vi "Configure Load to Sequence - ganged.vi"(8 "error in":errorcluster, 10 "measurement configuration":T6 {"Measurement timeout" format="%.3p"; "Load device voltage/current rating" format="%#_6pA"; "Load voltage/current setpoints" format="%#_6p"; "Load output function" items=["DC Voltage"=1006, "DC Current"=1007, "Pulse Voltage"=1049, "Pulse Current"=1050]; "Load sense" items=["Local"=1008, "Remote"=1009]; "Load transient response" items=["Slow"=1041, "Normal"=1038, "Fast"=1039, "Custom"=1042]; "Load current/voltage limit high" format="%#_6p"; "Load current/voltage limit low" format="%#_6p"; "Load current/voltage limit range" format="%#_6p"; "Load voltage/current level range" format="%#_6p"; "Power ON/Source voltage/current setpoints" format="%#_6p"; "Power ON/Source output function" items=["DC Voltage"=1006, "DC Current"=1007, "Pulse Voltage"=1049, "Pulse Current"=1050]; "Power ON/Source sense" items=["Local"=1008, "Remote"=1009]; "Source transient response" items=["Slow"=1041, "Normal"=1038, "Fast"=1039, "Custom"=1042]; "Source current/voltage limit high" format="%#_6p"; "Source current/voltage limit low" format="%#_6p"; "Power ON/Source current/voltage limit range" format="%#_6p"; "Source voltage/current level range" format="%#_6p"}, 11 "Waveform Mode - Control":T1={"Source Ganged Session Out"={"Ganged Config"=enum."Series", "Session List"=[], "Session Mode"=[], "Channel"=[]}, "Load Ganged Session Out"={"Ganged Config"=enum."Series", "Session List"=[], "Session Mode"=[], "Channel"=[]}, "Source Measure Record Length"=0, "Load Measure Record Length"=0, "Source Sequence Name"="", "Load Sequence Name"="", "Source First Sequence Call"=FALSE, "Load First Sequence Call"=FALSE, "Measurement Results"={"Source dt"=[], "Source voltages"=[], "Source currents"=[], "Ganged source voltages"=[], "Ganged source currents"=[0.0], "Load dt"=[], "Load voltages"=[], "Load currents"=[], "Ganged load voltages"=[], "Ganged load currents"=[], "Status"="", "Eload status"=""}, "No. of eload used"=0, "Measurement timeout"=0.0, "Load Source ON/OFF"=enum."SOURCE AND LOAD ON", "Load session out"="", "Source session out"="", "Load channel name"="", "Source channel name"="", "Source ganged/single"=FALSE, "Load ganged/single"=FALSE, "Source Master/Single resource name"="", "Source Slave resource name"=[], "Load Master/Single resource name"="", "Load Slave resource name"=[]}) -> (0 "error out":errorcluster, 3 "Waveform Mode - Result":T1={"Source Ganged Session Out"={"Ganged Config"=enum."Series", "Session List"=[], "Session Mode"=[], "Channel"=[]}, "Load Ganged Session Out"={"Ganged Config"=enum."Series", "Session List"=[], "Session Mode"=[], "Channel"=[]}, "Source Measure Record Length"=0, "Load Measure Record Length"=0, "Source Sequence Name"="", "Load Sequence Name"="", "Source First Sequence Call"=FALSE, "Load First Sequence Call"=FALSE, "Measurement Results"={"Source dt"=[], "Source voltages"=[], "Source currents"=[], "Ganged source voltages"=[], "Ganged source currents"=[0.0], "Load dt"=[], "Load voltages"=[], "Load currents"=[], "Ganged load voltages"=[], "Ganged load currents"=[], "Status"="", "Eload status"=""}, "No. of eload used"=0, "Measurement timeout"=0.0, "Load Source ON/OFF"=enum."SOURCE AND LOAD ON", "Load session out"="", "Source session out"="", "Load channel name"="", "Source channel name"="", "Source ganged/single"=FALSE, "Load ganged/single"=FALSE, "Source Master/Single resource name"="", "Source Slave resource name"=[], "Load Master/Single resource name"="", "Load Slave resource name"=[]})   [LabVIEW 2021, in "Waveform Mode_Channel Ganging.lvlib"]
doc: "Configures load ganged to sequence"
uses:
  Measurement Configuration.ctl
  Controls/Waveform Mode Measurement.ctl
  shared subVIs/ctl/NIDCPower_channel_ganging - ctl - ganged session.ctl
  shared subVIs/ctl/NIDCPower_channel_ganging - ctl - ganged config.ctl
  shared subVIs/ctl/NIDCPower_channel_ganging - ctl - channel mode.ctl
  Measurement Results.ctl
  <instrlib>/niDCPower/nidcpower.llb/niDCPower Source Mode.ctl
  <instrlib>/niDCPower/nidcpower.llb/niDCPower Sequence Attribute Type.ctl
  <instrlib>/niDCPower/nidcpower.llb/niDCPower Create Advanced Sequence Step With Channels.vi
  Waveform Mode_Channel Ganging.lvlib
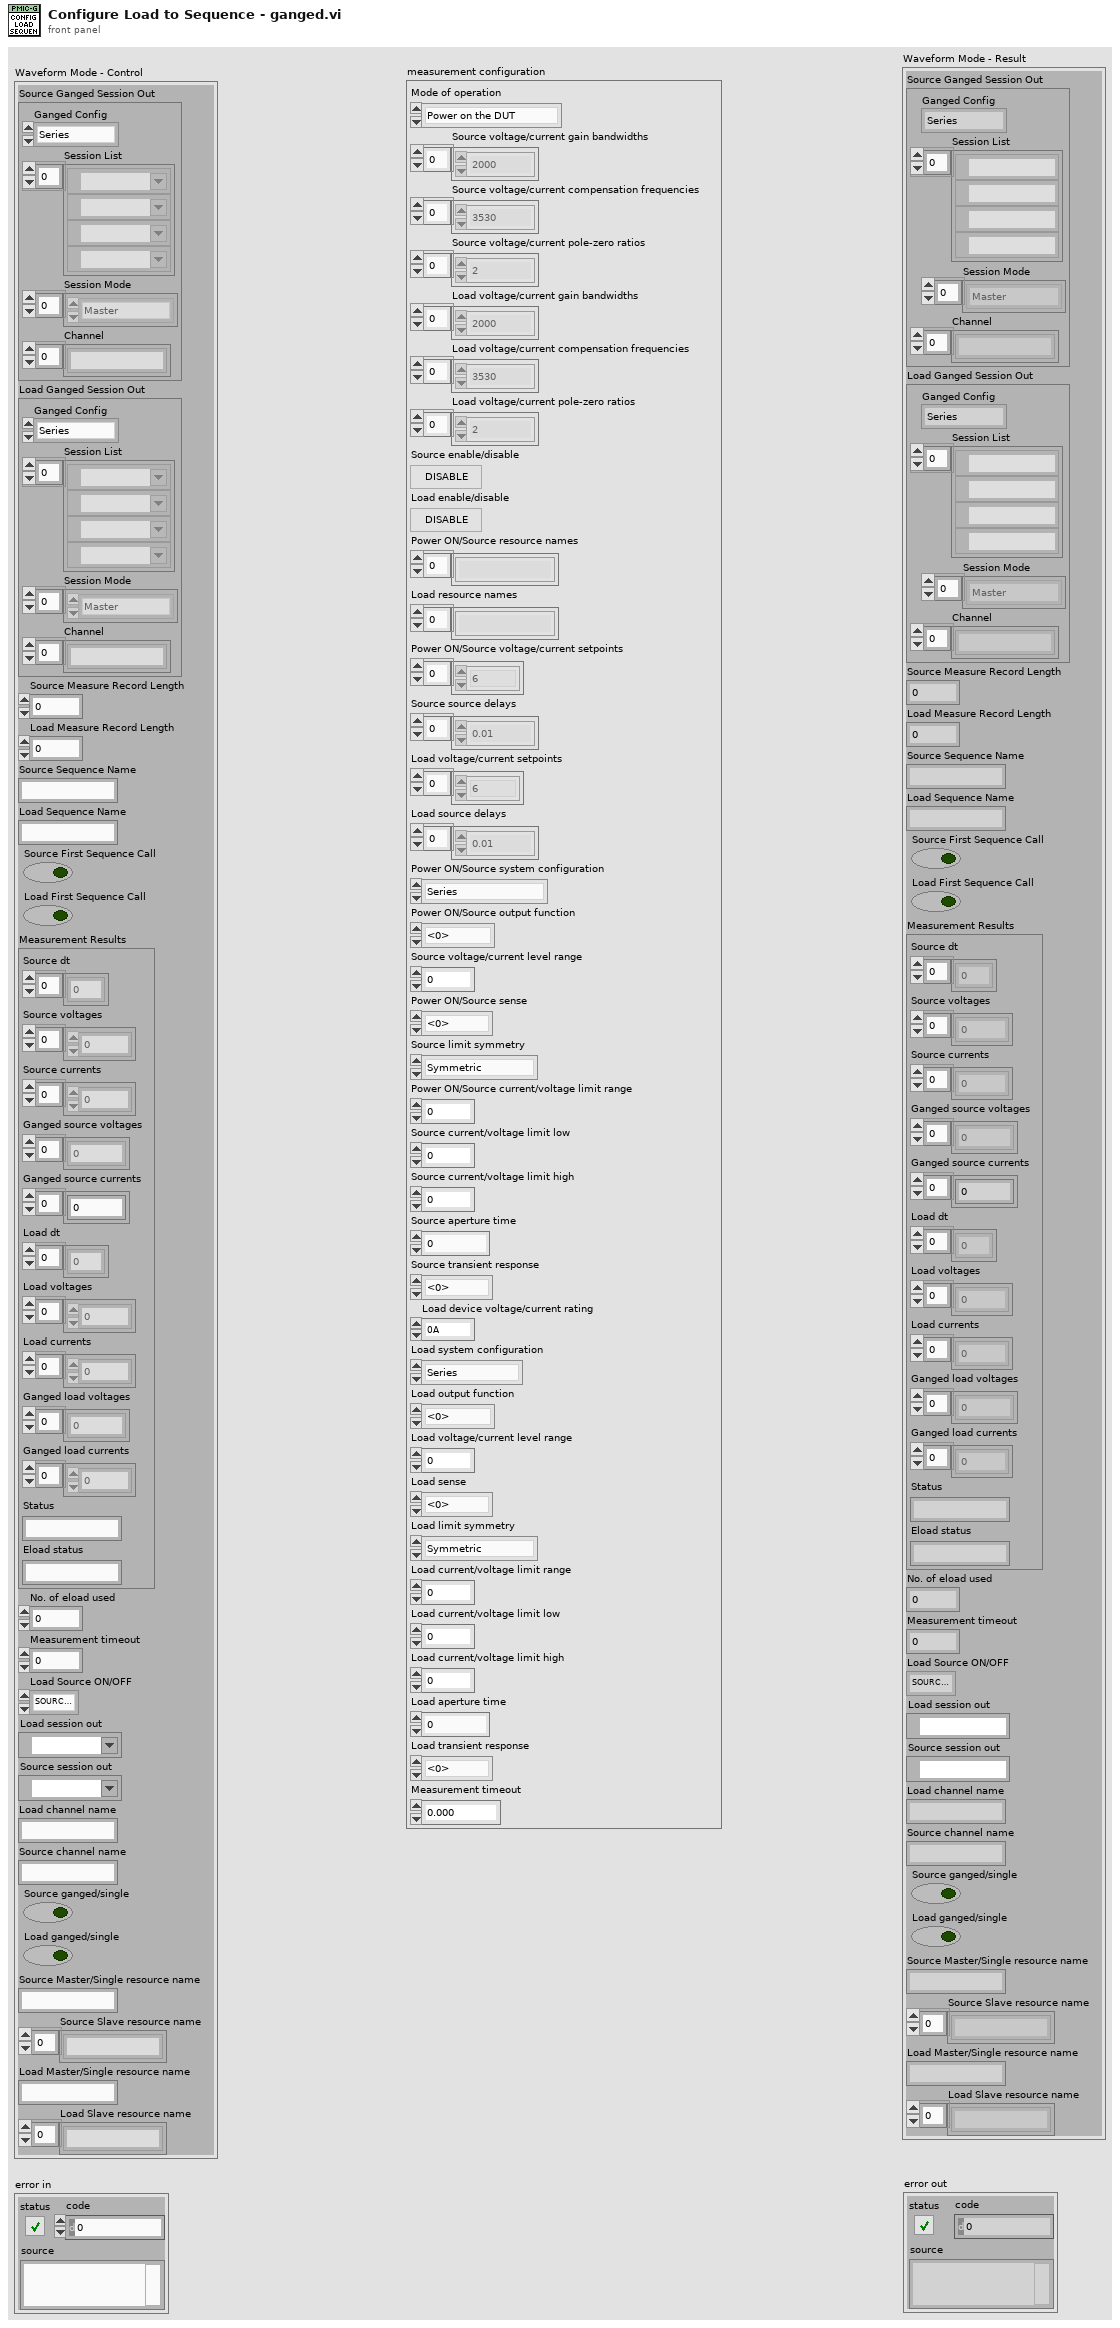
[diagram p1: front panel]
types:
  T1 = typedef "Waveform Mode_Channel Ganging.lvlib/Waveform Mode Measurement.ctl" = cluster{"Source Ganged Session Out":T2, "Load Ganged Session Out":T2, "Source Measure Record Length":i32, "Load Measure Record Length":i32, "Source Sequence Name":string, "Load Sequence Name":string, "Source First Sequence Call":bool, "Load First Sequence Call":bool, "Measurement Results":T5, "No. of eload used":i32, "Measurement timeout":dbl, "Load Source ON/OFF":enum16{"SOURCE AND LOAD OFF", "SOURCE ON", "LOAD ON", "SOURCE AND LOAD ON"}, "Load session out":refnum<k15>, "Source session out":refnum<k15>, "Load channel name":string, "Source channel name":string, "Source ganged/single":bool, "Load ganged/single":bool, "Source Master/Single resource name":string, "Source Slave resource name":string[], "Load Master/Single resource name":string, "Load Slave resource name":string[]}
  T2 = typedef "NIDCPower_channel_ganging - ctl - ganged session.ctl" = cluster{"Ganged Config":T3, "Session List":refnum<k15>[], "Session Mode":T4[], "Channel":string[]}
  T3 = typedef "NIDCPower_channel_ganging - ctl - ganged config.ctl" = enum32{"Series", "Parallel", "Manual"}
  T4 = typedef "NIDCPower_channel_ganging - ctl - channel mode.ctl" = enum32{"Master", "Slave", "Slave - Inverted"}
  T5 = typedef "Waveform Mode_Channel Ganging.lvlib/Measurement Results.ctl" = cluster{"Source dt":dbl[], "Source voltages":dbl[], "Source currents":dbl[], "Ganged source voltages":dbl[], "Ganged source currents":dbl[], "Load dt":dbl[], "Load voltages":dbl[], "Load currents":dbl[], "Ganged load voltages":dbl[], "Ganged load currents":dbl[], "Status":string, "Eload status":string}
  T6 = typedef "Waveform Mode_Channel Ganging.lvlib/Measurement Configuration.ctl" = cluster{"Mode of operation":enum32{"Power on the DUT", "Perform measurement", "Power off the DUT"}, "Source voltage/current gain bandwidths":dbl[], "Source voltage/current compensation frequencies":dbl[], "Source voltage/current pole-zero ratios":dbl[], "Load voltage/current gain bandwidths":dbl[], "Load voltage/current compensation frequencies":dbl[], "Load voltage/current pole-zero ratios":dbl[], "Source enable/disable":bool, "Load enable/disable":bool, "Power ON/Source resource names":string[], "Load resource names":string[], "Power ON/Source voltage/current setpoints":dbl[], "Source source delays":dbl[], "Load voltage/current setpoints":dbl[], "Load source delays":dbl[], "Power ON/Source system configuration":enum32{"Series", "Parallel", "Manual"}, "Power ON/Source output function":i32, "Source voltage/current level range":dbl, "Power ON/Source sense":i32, "Source limit symmetry":enum32{"Symmetric", "Asymmetric"}, "Power ON/Source current/voltage limit range":dbl, "Source current/voltage limit low":dbl, "Source current/voltage limit high":dbl, "Source aperture time":dbl, "Source transient response":i32, "Load device voltage/current rating":dbl, "Load system configuration":enum32{"Series", "Parallel", "Manual"}, "Load output function":i32, "Load voltage/current level range":dbl, "Load sense":i32, "Load limit symmetry":enum32{"Symmetric", "Asymmetric"}, "Load current/voltage limit range":dbl, "Load current/voltage limit low":dbl, "Load current/voltage limit high":dbl, "Load aperture time":dbl, "Load transient response":i32, "Measurement timeout":dbl}
  T7 = typedef "niDCPower Source Mode.ctl" = i32
  T8 = typedef "niDCPower Sequence Attribute Type.ctl" = i32
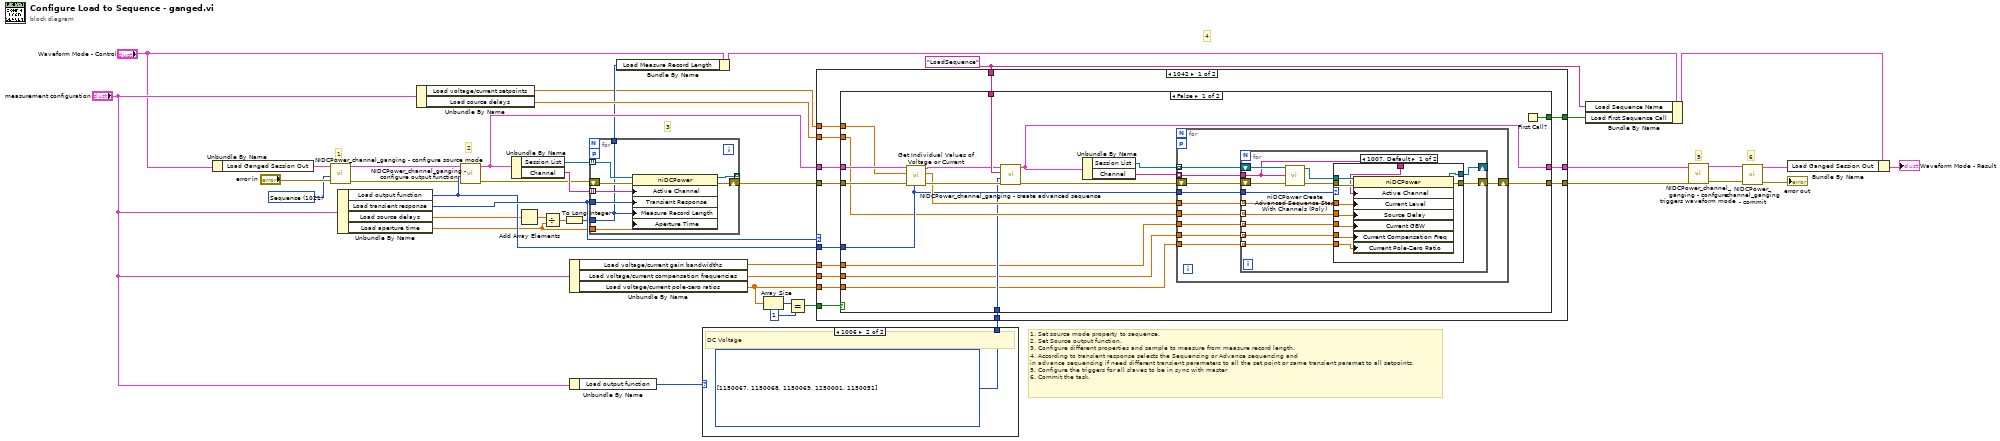
[diagram p0: block diagram]
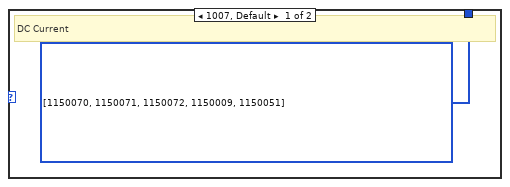
[diagram p2: hidden frame]
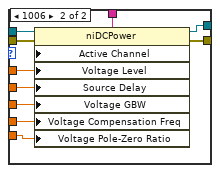
[diagram p3: hidden frame]
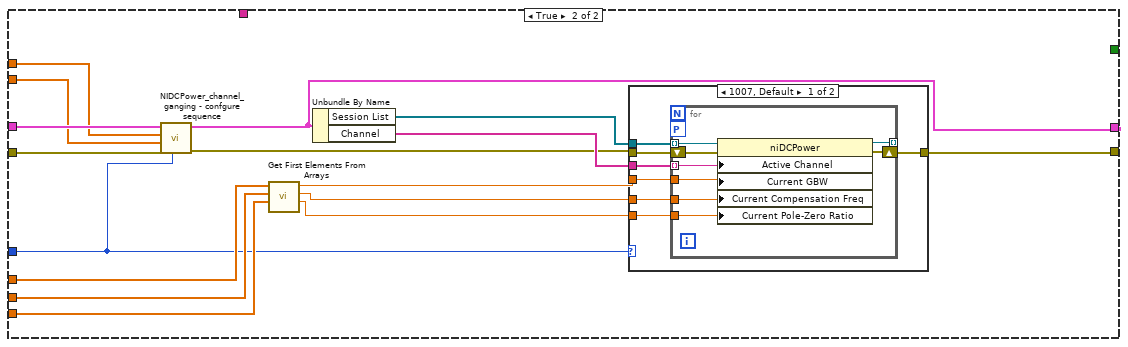
[diagram p4: hidden frame]
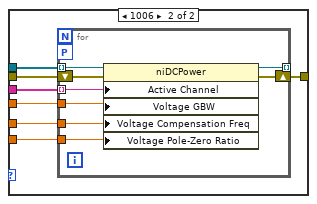
[diagram p5: hidden frame]
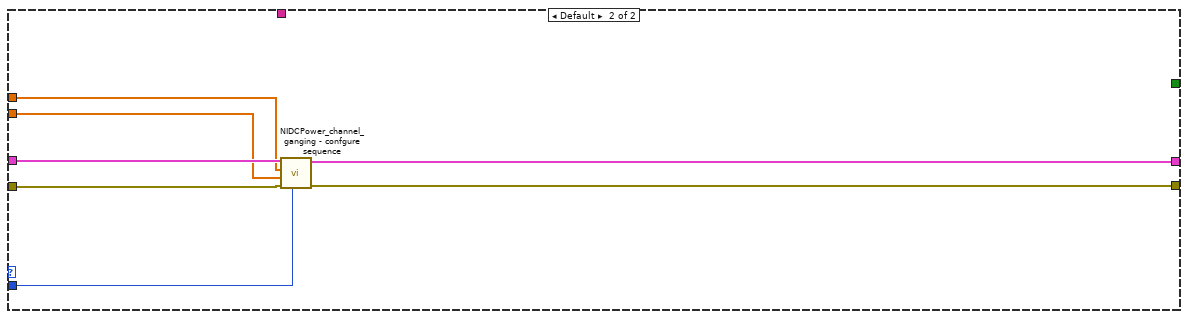
[diagram p6: hidden frame]
diagram:
  w32 = "LoadSequence" ("sequence name")
  w5 = T7 1021 items=["Single Point"=1020, "Sequence"=1021] ("source mode")
  # "1. Set source mode property to sequence.\n2. Set Source output function.\n3. Configure different properties and sample to measure from measure record length.\n4. According to transient response selects the Sequencing or Advance sequencing and\nin advance sequencing if need different transient parameters to all the set point or same transient paramet to all setpoints.\n5. Configure the triggers for all slaves to be in sync with master\n6. Commit the task."
  # "1. Set source mode property to sequence.\n2. Set Source output function.\n3. Configure different properties and sample to measure from measure record length.\n4. According to transient response selects the Sequencing or Advance sequencing and\nin advance sequencing if need different transient parameters to all the set point or same transient paramet to all setpoints.\n5. Configure the triggers for all slaves to be in sync with master\n6. Commit the task."
  # "6"
  # "5"
  # "4"
  # "3"
  # "2"
  # "1"
  n1 = Unbundle By Name("Waveform Mode - Control") -> ("Load Ganged Session Out"=w9:T2)
  n2 = call "NIDCPower_channel_ganging - configure source mode.vi"("error in (no error)"="error in", "source mode"=w5, "Ganged Session In"=w9) -> ("error out"=w3:errorcluster, "Ganged Session Out"=w4:T2)  [unwired: 7 in]
  n3 = Unbundle By Name("measurement configuration") -> ("Load output function"=w29:i32, "Load transient response"=w30:i32, "Load source delays"=w15:dbl[], "Load aperture time"=w17:dbl)
  n4 = Unbundle By Name("measurement configuration") -> ("Load voltage/current setpoints"=w11:dbl[], "Load source delays"=w20:dbl[])
  n5 = call "NIDCPower_channel_ganging - configure output function.vi"("error in (no error)"=w3, "output function"=w29, "Ganged Session In"=w4) -> ("error out"=w6:errorcluster, "Ganged Session Out"=w19:T2)  [unwired: 7 in]
  n6 = Unbundle By Name(w19) -> ("Session List"=w7:refnum<k15>[], "Channel"=w10:string[])
  n7 = Add Array Elements(numeric array=w15) -> (sum=w12:dbl)
  n8 = Divide(x=w12, y=w17) -> (x/y=w13:dbl)
  n9 = To Long Integer(number=w13) -> (32bit integer=w14:i32)
  n10 = Unbundle By Name("measurement configuration") -> ("Load voltage/current gain bandwidths"=w21:dbl[], "Load voltage/current compensation frequencies"=w22:dbl[], "Load voltage/current pole-zero ratios"=w28:dbl[])
  n11 = Unbundle By Name("measurement configuration") -> ("Load output function"=w35:i32)
  n12 = for {
    tunnel: [w49] -> _ mode=indexing
    shift-right: [w47] -> w18
    shift-left: w6 -> [w48]
    workers-P: _ -> [_]
    tunnel: w7 -> [w46] mode=indexing
    tunnel: w10 -> [w45] mode=indexing
    tunnel: w30 -> [w44]
    tunnel: w17 -> [w43]
    tunnel: w14 -> [w42]
    tunnel: [w42] -> w16
    n13 = property class="niDCPower"(reference=w46, error in=w48, "Active Channel"=w45, "Transient Response"=w44, "Measure Record Length"=w42, "Aperture Time"=w43) -> (reference out=w49:refnum<k15>, error out=w47:errorcluster)
  }
  n14 = Bundle By Name(cluster="Waveform Mode - Control", "Load Measure Record Length"=w16) -> (w41:T1)
  n15 = case shown="1006" w35 {
    tunnel: [w50 w51] -> w33
    frame 1007, Default {
      w50 = T8[] [1150070, 1150071, 1150072, 1150009, 1150051] items=["Source -> Output Function"=1150008, "Source -> Output Enabled"=1250006, "Source -> Output Resistance"=1150061, "Source -> Transient Response"=1150062, "Source -> Custom Transient Response -> Voltage Gain Bandwidth"=1150067, "Source -> Custom Transient Response -> Voltage Compensation Frequency"=1150068, "Source -> Custom Transient Response -> Voltage Pole-Zero Ratio"=1150069, "Source -> Custom Transient Response -> Current Gain Bandwidth"=1150070, "Source -> Custom Transient Response -> Current Compensation Frequency"=1150071, "Source -> Custom Transient Response -> Current Pole-Zero Ratio"=1150072, "Source -> DC Voltage -> Voltage Level"=1250001, "Source -> DC Voltage -> Voltage Level Range"=1150005, "Source -> DC Voltage -> Current Limit"=1250005, "Source -> DC Voltage -> Current Limit High"=1150187, "Source -> DC Voltage -> Current Limit Low"=1150188, "Source -> DC Voltage -> Current Limit Range"=1150004, "Source -> DC Current -> Current Level"=1150009, "Source -> DC Current -> Current Level Range"=1150011, "Source -> DC Current -> Voltage Limit"=1150010, "Source -> DC Current -> Voltage Limit High"=1150185, "Source -> DC Current -> Voltage Limit Low"=1150186, "Source -> DC Current -> Voltage Limit Range"=1150012, "Source -> DC Current -> Current Level Slew Rate -> Rising"=1150343, "Source -> DC Current -> Current Level Slew Rate -> Falling"=1150344, "Source -> Pulse Voltage -> Pulse Voltage Level"=1150080, "Source -> Pulse Voltage -> Pulse Bias Voltage Level"=1150082, "Source -> Pulse Voltage -> Pulse Voltage Level Range"=1150084, "Source -> Pulse Voltage -> Pulse Current Limit"=1150081, "Source -> Pulse Voltage -> Pulse Current Limit High"=1150193, "Source -> Pulse Voltage -> Pulse Current Limit Low"=1150194, "Source -> Pulse Voltage -> Pulse Bias Current Limit"=1150083, "Source -> Pulse Voltage -> Pulse Bias Current Limit High"=1150195, "Source -> Pulse Voltage -> Pulse Bias Current Limit Low"=1150196, "Source -> Pulse Voltage -> Pulse Current Limit Range"=1150085, "Source -> Pulse Current -> Pulse Current Level"=1150086, "Source -> Pulse Current -> Pulse Bias Current Level"=1150088, "Source -> Pulse Current -> Pulse Current Level Range"=1150090, "Source -> Pulse Current -> Pulse Voltage Limit"=1150087, "Source -> Pulse Current -> Pulse Voltage Limit High"=1150189, "Source -> Pulse Current -> Pulse Voltage Limit Low"=1150190, "Source -> Pulse Current -> Pulse Bias Voltage Limit"=1150089, "Source -> Pulse Current -> Pulse Bias Voltage Limit High"=1150191, "Source -> Pulse Current -> Pulse Bias Voltage Limit Low"=1150192, "Source -> Pulse Current -> Pulse Voltage Limit Range"=1150091, "Source -> Advanced -> Source Delay"=1150051, "Source -> Advanced -> Pulse Bias Delay"=1150092, "Source -> Advanced -> Pulse On Time"=1150093, "Source -> Advanced -> Pulse Off Time"=1150094, "Source -> Advanced -> OVP Enabled"=1250002, "Source -> Advanced -> OVP Limit"=1250003, "Source -> Advanced -> Compliance Limit Symmetry"=1150184, "Source -> Advanced -> Sequence Step Delta Time"=1150198, "Source -> Advanced -> Conduction Voltage -> Mode"=1150350, "Source -> Advanced -> Conduction Voltage -> On Threshold"=1150351, "Source -> Advanced -> Conduction Voltage -> Off Threshold"=1150352, "Measurement -> Sense"=1150013, "Measurement -> Aperture Time"=1150058, "Measurement -> Measure Record Length"=1150063, "Measurement -> Advanced -> DC Noise Rejection"=1150066, "Measurement -> Autorange"=1150244, "Measurement -> Advanced -> Autorange Behavior"=1150245, "Measurement -> Advanced -> Autorange Aperture Time Mode"=1150246, "Measurement -> Advanced -> Autorange Minimum Aperture Time"=1150247, "Measurement -> Advanced -> Autorange Minimum Aperture Time Units"=1150248, "Measurement -> Advanced -> Autorange Minimum Current Range"=1150255, "Measurement -> Advanced -> Autorange Minimum Voltage Range"=1150256, "Measurement -> Advanced -> Autorange Threshold Mode"=1150257, "Measurement -> Advanced -> Autorange Maximum Delay After Range Change"=1150322, "LCR -> Instrument Mode"=1150208, "LCR -> Source Delay Mode"=1150315, "LCR -> Measurement Time"=1150218, "LCR -> Custom Measurement Time"=1150258, "LCR -> AC Stimulus -> Function"=1150209, "LCR -> AC Stimulus -> Frequency"=1150210, "LCR -> AC Stimulus -> Voltage Amplitude"=1150211, "LCR -> AC Stimulus -> Current Amplitude"=1150212, "LCR -> AC Stimulus -> Advanced -> Voltage Range"=1150265, "LCR -> AC Stimulus -> Advanced -> Current Range"=1150267, "LCR -> AC Stimulus -> Advanced -> Source Aperture Time"=1150349, "LCR -> DC Bias -> Source"=1150213, "LCR -> DC Bias -> Voltage Level"=1150214, "LCR -> DC Bias -> Current Level"=1150215, "LCR -> DC Bias -> Advanced -> Voltage Range"=1150266, "LCR -> DC Bias -> Advanced -> Current Range"=1150274, "LCR -> DC Bias -> Advanced -> Transient Response"=1150347, "LCR -> Compensation -> Open -> Enabled"=1150220, "LCR -> Compensation -> Open -> Conductance"=1150261, "LCR -> Compensation -> Open -> Susceptance"=1150262, "LCR -> Compensation -> Short -> Enabled"=1150221, "LCR -> Compensation -> Short -> Resistance"=1150263, "LCR -> Compensation -> Short -> Reactance"=1150264, "LCR -> Compensation -> Load -> Enabled"=1150222, "LCR -> Compensation -> Load -> Measured Resistance"=1150268, "LCR -> Compensation -> Load -> Measured Reactance"=1150269, "LCR -> Compensation -> Load -> Actual Resistance"=1150270, "LCR -> Compensation -> Load -> Actual Reactance"=1150271, "LCR -> Impedance Range -> Impedance Range"=1150217, "LCR -> Impedance Range -> Impedance Autorange"=1150216, "LCR -> Impedance Range -> Advanced -> Impedance Range Source"=1150321, "LCR -> Impedance Range -> Advanced -> Load Resistance"=1150318, "LCR -> Impedance Range -> Advanced -> Load Inductance"=1150319, "LCR -> Impedance Range -> Advanced -> Load Capacitance"=1150320] ("advanced sequence properties")
      # "DC Current"
    }
    frame 1006 {
      w51 = T8[] [1150067, 1150068, 1150069, 1250001, 1150051] items=["Source -> Output Function"=1150008, "Source -> Output Enabled"=1250006, "Source -> Output Resistance"=1150061, "Source -> Transient Response"=1150062, "Source -> Custom Transient Response -> Voltage Gain Bandwidth"=1150067, "Source -> Custom Transient Response -> Voltage Compensation Frequency"=1150068, "Source -> Custom Transient Response -> Voltage Pole-Zero Ratio"=1150069, "Source -> Custom Transient Response -> Current Gain Bandwidth"=1150070, "Source -> Custom Transient Response -> Current Compensation Frequency"=1150071, "Source -> Custom Transient Response -> Current Pole-Zero Ratio"=1150072, "Source -> DC Voltage -> Voltage Level"=1250001, "Source -> DC Voltage -> Voltage Level Range"=1150005, "Source -> DC Voltage -> Current Limit"=1250005, "Source -> DC Voltage -> Current Limit High"=1150187, "Source -> DC Voltage -> Current Limit Low"=1150188, "Source -> DC Voltage -> Current Limit Range"=1150004, "Source -> DC Current -> Current Level"=1150009, "Source -> DC Current -> Current Level Range"=1150011, "Source -> DC Current -> Voltage Limit"=1150010, "Source -> DC Current -> Voltage Limit High"=1150185, "Source -> DC Current -> Voltage Limit Low"=1150186, "Source -> DC Current -> Voltage Limit Range"=1150012, "Source -> DC Current -> Current Level Slew Rate -> Rising"=1150343, "Source -> DC Current -> Current Level Slew Rate -> Falling"=1150344, "Source -> Pulse Voltage -> Pulse Voltage Level"=1150080, "Source -> Pulse Voltage -> Pulse Bias Voltage Level"=1150082, "Source -> Pulse Voltage -> Pulse Voltage Level Range"=1150084, "Source -> Pulse Voltage -> Pulse Current Limit"=1150081, "Source -> Pulse Voltage -> Pulse Current Limit High"=1150193, "Source -> Pulse Voltage -> Pulse Current Limit Low"=1150194, "Source -> Pulse Voltage -> Pulse Bias Current Limit"=1150083, "Source -> Pulse Voltage -> Pulse Bias Current Limit High"=1150195, "Source -> Pulse Voltage -> Pulse Bias Current Limit Low"=1150196, "Source -> Pulse Voltage -> Pulse Current Limit Range"=1150085, "Source -> Pulse Current -> Pulse Current Level"=1150086, "Source -> Pulse Current -> Pulse Bias Current Level"=1150088, "Source -> Pulse Current -> Pulse Current Level Range"=1150090, "Source -> Pulse Current -> Pulse Voltage Limit"=1150087, "Source -> Pulse Current -> Pulse Voltage Limit High"=1150189, "Source -> Pulse Current -> Pulse Voltage Limit Low"=1150190, "Source -> Pulse Current -> Pulse Bias Voltage Limit"=1150089, "Source -> Pulse Current -> Pulse Bias Voltage Limit High"=1150191, "Source -> Pulse Current -> Pulse Bias Voltage Limit Low"=1150192, "Source -> Pulse Current -> Pulse Voltage Limit Range"=1150091, "Source -> Advanced -> Source Delay"=1150051, "Source -> Advanced -> Pulse Bias Delay"=1150092, "Source -> Advanced -> Pulse On Time"=1150093, "Source -> Advanced -> Pulse Off Time"=1150094, "Source -> Advanced -> OVP Enabled"=1250002, "Source -> Advanced -> OVP Limit"=1250003, "Source -> Advanced -> Compliance Limit Symmetry"=1150184, "Source -> Advanced -> Sequence Step Delta Time"=1150198, "Source -> Advanced -> Conduction Voltage -> Mode"=1150350, "Source -> Advanced -> Conduction Voltage -> On Threshold"=1150351, "Source -> Advanced -> Conduction Voltage -> Off Threshold"=1150352, "Measurement -> Sense"=1150013, "Measurement -> Aperture Time"=1150058, "Measurement -> Measure Record Length"=1150063, "Measurement -> Advanced -> DC Noise Rejection"=1150066, "Measurement -> Autorange"=1150244, "Measurement -> Advanced -> Autorange Behavior"=1150245, "Measurement -> Advanced -> Autorange Aperture Time Mode"=1150246, "Measurement -> Advanced -> Autorange Minimum Aperture Time"=1150247, "Measurement -> Advanced -> Autorange Minimum Aperture Time Units"=1150248, "Measurement -> Advanced -> Autorange Minimum Current Range"=1150255, "Measurement -> Advanced -> Autorange Minimum Voltage Range"=1150256, "Measurement -> Advanced -> Autorange Threshold Mode"=1150257, "Measurement -> Advanced -> Autorange Maximum Delay After Range Change"=1150322, "LCR -> Instrument Mode"=1150208, "LCR -> Source Delay Mode"=1150315, "LCR -> Measurement Time"=1150218, "LCR -> Custom Measurement Time"=1150258, "LCR -> AC Stimulus -> Function"=1150209, "LCR -> AC Stimulus -> Frequency"=1150210, "LCR -> AC Stimulus -> Voltage Amplitude"=1150211, "LCR -> AC Stimulus -> Current Amplitude"=1150212, "LCR -> AC Stimulus -> Advanced -> Voltage Range"=1150265, "LCR -> AC Stimulus -> Advanced -> Current Range"=1150267, "LCR -> AC Stimulus -> Advanced -> Source Aperture Time"=1150349, "LCR -> DC Bias -> Source"=1150213, "LCR -> DC Bias -> Voltage Level"=1150214, "LCR -> DC Bias -> Current Level"=1150215, "LCR -> DC Bias -> Advanced -> Voltage Range"=1150266, "LCR -> DC Bias -> Advanced -> Current Range"=1150274, "LCR -> DC Bias -> Advanced -> Transient Response"=1150347, "LCR -> Compensation -> Open -> Enabled"=1150220, "LCR -> Compensation -> Open -> Conductance"=1150261, "LCR -> Compensation -> Open -> Susceptance"=1150262, "LCR -> Compensation -> Short -> Enabled"=1150221, "LCR -> Compensation -> Short -> Resistance"=1150263, "LCR -> Compensation -> Short -> Reactance"=1150264, "LCR -> Compensation -> Load -> Enabled"=1150222, "LCR -> Compensation -> Load -> Measured Resistance"=1150268, "LCR -> Compensation -> Load -> Measured Reactance"=1150269, "LCR -> Compensation -> Load -> Actual Resistance"=1150270, "LCR -> Compensation -> Load -> Actual Reactance"=1150271, "LCR -> Impedance Range -> Impedance Range"=1150217, "LCR -> Impedance Range -> Impedance Autorange"=1150216, "LCR -> Impedance Range -> Advanced -> Impedance Range Source"=1150321, "LCR -> Impedance Range -> Advanced -> Load Resistance"=1150318, "LCR -> Impedance Range -> Advanced -> Load Inductance"=1150319, "LCR -> Impedance Range -> Advanced -> Load Capacitance"=1150320] ("advanced sequence properties")
      # "DC Voltage"
    }
  }
  n16 = Array Size(array=w28) -> (size(s)=w25:i32)
  n17 = Equal?(x=w25, y=1) -> (x = y?=w27:bool)
  n18 = case shown="1042" w30 {
    tunnel: w19 -> [w58 w180]
    tunnel: [w64 w179] -> w24
    tunnel: [w65 w178] -> w23
    tunnel: w11 -> [w57 w176]
    tunnel: w18 -> [w59 w177]
    tunnel: w20 -> [w53 w175]
    tunnel: w21 -> [w63 _]
    tunnel: w22 -> [w62 _]
    tunnel: w28 -> [w61 _]
    tunnel: w32 -> [w60 _]
    tunnel: w27 -> [w56 _]
    tunnel: w29 -> [w55 w174]
    tunnel: [w54 _] -> w31
    tunnel: w33 -> [w52 _]
    frame 1042 {
      n19 = case shown="False" w56 {
        tunnel: [w84 w141] -> w65
        tunnel: [w83 w128] -> w64
        tunnel: w63 -> [w68 w137]
        tunnel: w62 -> [w67 w136]
        tunnel: w61 -> [w66 w135]
        tunnel: w60 -> [w79 _]
        tunnel: w59 -> [w76 w134]
        tunnel: w58 -> [w75 w132]
        tunnel: w57 -> [w74 w130]
        tunnel: w55 -> [w72 w131]
        tunnel: [w71 _] -> w54
        tunnel: w53 -> [w70 w129]
        tunnel: w52 -> [w69 _]
        frame False {
          n20 = call "Get Individual Values of Voltage or Current.vi"("output function"=w72, "error in (no error)"=w76, "Values In"=w74, "Ganged Session In"=w75) -> ("error out"=w77:errorcluster, "Values Out"=w73:dbl[], "Ganged Session Out"=w78:T2)  [unwired: 5 in]
          n21 = call "NIDCPower_channel_ganging - create advanced sequence.vi"("error in (no error)"=w77, "advanced sequence properties"=w69, "sequence name"=w79, "Ganged Session In"=w78) -> ("error out"=w81:errorcluster, "Ganged Session Out"=w83:T2)  [unwired: 6 in]
          n22 = Unbundle By Name(w83) -> ("Session List"=w82:refnum<k15>[], "Channel"=w80:string[])
          n23 = for {
            workers-P: _ -> [_]
            tunnel: w82 -> [w94] mode=indexing
            shift-right: [w92] -> w84
            shift-left: w81 -> [w93]
            tunnel: w80 -> [w91] mode=indexing
            tunnel: w73 -> [w90]
            tunnel: w66 -> [w89]
            tunnel: w68 -> [w88]
            tunnel: w67 -> [w87]
            tunnel: w70 -> [w86]
            tunnel: w72 -> [w85]
            n24 = for {
              shift-right: [w102] -> _
              shift-left: w94 -> [w107]
              shift-right: [w101] -> w92
              shift-left: w93 -> [w106]
              tunnel: w91 -> [w104]
              tunnel: w90 -> [w103] mode=indexing
              tunnel: w89 -> [w96] mode=indexing
              tunnel: w88 -> [w98] mode=indexing
              tunnel: w87 -> [w97] mode=indexing
              tunnel: w86 -> [w99] mode=indexing
              tunnel: w85 -> [w95]
              n25 = call-poly <instrlib>:"niDCPower Create Advanced Sequence Step With Channels (Poly).vi"("error in (no error)"=w106, "channel name"=w104, "instrument handle"=w107) -> ("error out"=w100:errorcluster, "instrument handle out"=w105:refnum<k15>)  [unwired: 7 in]
              n26 = case shown="1007, Default" w95 {
                tunnel: w105 -> [w117 w127]
                tunnel: w104 -> [w113 w126]
                tunnel: w103 -> [w112 w125]
                tunnel: [w114 w124] -> w102
                tunnel: [w115 w123] -> w101
                tunnel: w100 -> [w116 w122]
                tunnel: w99 -> [w111 w121]
                tunnel: w98 -> [w110 w120]
                tunnel: w97 -> [w109 w119]
                tunnel: w96 -> [w108 w118]
                frame 1007, Default {
                  n27 = property class="niDCPower"(reference=w117, error in=w116, "Active Channel"=w113, "Current Level"=w112, "Source Delay"=w111, "Current GBW"=w110, "Current Compensation Freq"=w109, "Current Pole-Zero Ratio"=w108) -> (reference out=w114:refnum<k15>, error out=w115:errorcluster)
                }
                frame 1006 {
                  n28 = property class="niDCPower"(reference=w127, error in=w122, "Active Channel"=w126, "Voltage Level"=w125, "Source Delay"=w121, "Voltage GBW"=w120, "Voltage Compensation Freq"=w119, "Voltage Pole-Zero Ratio"=w118) -> (reference out=w124:refnum<k15>, error out=w123:errorcluster)
                }
              }
            }
          }
          n29 = First Call?() -> (First Call?: T/F=w71:bool)
        }
        frame True {
          n30 = call "NIDCPower_channel_ganging - confgure sequence.vi"("output function"=w131, "error in (no error)"=w134, "Source Delays"=w129, "Values"=w130, "Ganged Session In"=w132) -> ("error out"=w133:errorcluster, "Ganged Session Out"=w128:T2)  [unwired: 5 in]
          n31 = call "Get First Elements From Arrays.vi"("Pole-zero ratios"=w135, "Compensation frequencies"=w136, "Gain bandwidths"=w137) -> ("Pole-zero ratio"=w138:dbl, "Compensation frequency"=w139:dbl, "Gain bandwidth"=w140:dbl)  [unwired: 6 in]
          n32 = Unbundle By Name(w128) -> ("Session List"=w143:refnum<k15>[], "Channel"=w142:string[])
          n33 = case shown="1007, Default" w131 {
            tunnel: w133 -> [w150 w165]
            tunnel: [w149 w164] -> w141
            tunnel: w143 -> [w148 w163]
            tunnel: w142 -> [w146 w162]
            tunnel: w140 -> [w147 w161]
            tunnel: w138 -> [w144 w159]
            tunnel: w139 -> [w145 w160]
            frame 1007, Default {
              n34 = for {
                workers-P: _ -> [_]
                shift-right: [w157] -> w149
                shift-left: w150 -> [w158]
                tunnel: w148 -> [w156] mode=indexing
                tunnel: [w155] -> _ mode=indexing
                tunnel: w147 -> [w154]
                tunnel: w146 -> [w153] mode=indexing
                tunnel: w145 -> [w152]
                tunnel: w144 -> [w151]
                n35 = property class="niDCPower"(reference=w156, error in=w158, "Active Channel"=w153, "Current GBW"=w154, "Current Compensation Freq"=w152, "Current Pole-Zero Ratio"=w151) -> (reference out=w155:refnum<k15>, error out=w157:errorcluster)
              }
            }
            frame 1006 {
              n36 = for {
                workers-P: _ -> [_]
                shift-right: [w166] -> w164
                shift-left: w165 -> [w173]
                tunnel: w163 -> [w172] mode=indexing
                tunnel: [w171] -> _ mode=indexing
                tunnel: w162 -> [w170] mode=indexing
                tunnel: w161 -> [w169]
                tunnel: w160 -> [w168]
                tunnel: w159 -> [w167]
                n37 = property class="niDCPower"(reference=w172, error in=w173, "Active Channel"=w170, "Voltage GBW"=w169, "Voltage Compensation Freq"=w168, "Voltage Pole-Zero Ratio"=w167) -> (reference out=w171:refnum<k15>, error out=w166:errorcluster)
              }
            }
          }
        }
      }
    }
    frame Default {
      n38 = call "NIDCPower_channel_ganging - confgure sequence.vi"("output function"=w174, "error in (no error)"=w177, "Source Delays"=w175, "Values"=w176, "Ganged Session In"=w180) -> ("error out"=w178:errorcluster, "Ganged Session Out"=w179:T2)  [unwired: 5 in]
    }
  }
  n39 = Bundle By Name(cluster=w41, "Load Sequence Name"=w32, "Load First Sequence Call"=w31) -> (w36:T1)
  n40 = call "NIDCPower_channel_ganging - confgure triggers waveform mode.vi"("error in (no error)"=w23, "Ganged Session in"=w24) -> ("error out"=w39:errorcluster, "Ganged Session out"=w37:T2)  [unwired: 8 in]
  n41 = call "NIDCPower_channel_ganging - commit.vi"("error in (no error)"=w39, "Ganged Session In"=w37) -> ("error out"=→"error out":errorcluster, "Ganged Session Out"=w38:T2)  [unwired: 8 in]
  n42 = Bundle By Name(cluster=w36, "Load Ganged Session Out"=w38) -> (→"Waveform Mode - Result":T1)
